vi "Bridge Lower Auto.vi"(9 "d":dbl) -> ()   [LabVIEW 2011]
uses:
  <vilib>/Rock Robotics/WPI/Solenoid/WPI_SolenoidValue.ctl
  <vilib>/Rock Robotics/WPI/Solenoid/WPI_SolenoidSetEnum.vi
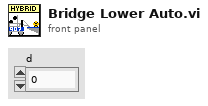
[diagram p1: front panel]
types:
  T1 = typedef "WPI_RobotDriveDevRef.ctl" = cluster{"DevStatus":errorcluster, "Motors[]":T2[], "Square Inputs":bool, "Max Output":dbl, "Isochronous":bool}
  T2 = typedef "WPI_MotorControlDeviceRef.ctl" = cluster{"DeviceStatus":errorcluster, "Type":enum16{"PWM", "CAN"}, "PWM":cluster{"Digital Module":T3, "PWM Channel":T4, "DeadBand":T5}, "CAN":cluster{"Device Number":u8, "Control Mode":T6, "Semaphore":T7, "Max Vout":dbl}, "Invert":bool, "TransformRef":T8, "InvTransformRef":T8}
  T3 = typedef "FPGA_TypedefDigitalModule.ctl" = enum16{"Digital Module 1", "Digital Module 2"}
  T4 = typedef "FPGA_DIOPWMChannel.ctl" = enum8{"PWM 1", "PWM 2", "PWM 3", "PWM 4", "PWM 5", "PWM 6", "PWM 7", "PWM 8", "PWM 9", "PWM 10", "Invalid"}
  T5 = typedef "WPI_PWMDeadband.ctl" = cluster{"Name":string, "maxPositivePwm":i32, "minPositivePwm":i32, "centerPwm":i32, "maxNegativePwm":i32, "minNegativePwm":i32, "angularRange":u16}
  T6 = typedef "WPI_CANJaguar_ControlMode.ctl" = enum8{"Percent VBus", "Current", "Speed", "Position", "Voltage"}
  T7 = typedef "Semaphore RefNum" = refnum<k1>
  T8 = typedef "WPI_PWMTransform_ConPane.ctl" = refnum<vi>
  T9 = typedef "WPI_SolenoidDevRef.ctl" = cluster{"DevStatus":errorcluster, "Solenoid Module":T10, "Forward Solenoid Channel":T11, "Reverse Solenoid Channel":T11}
  T10 = typedef "FPGA_TypedefSolenoidModule.ctl" = enum16{"Solenoid Module 1", "Solenoid Module 2"}
  T11 = typedef "WPI_SolenoidChannel.ctl" = enum8{"Solenoid 1", "Solenoid 2", "Solenoid 3", "Solenoid 4", "Solenoid 5", "Solenoid 6", "Solenoid 7", "Solenoid 8", "Invalid"}
  T12 = typedef "WPI_EncoderDevRef.ctl" = cluster{"DevStatus":errorcluster, "EncoderIndex":T13, "CounterIndex":T14, "DistancePerCount":dbl, "Decoding Type":T15}
  T13 = typedef "FPGA_EncoderIdx.ctl" = enum8{"Enc 0", "Enc 1", "Enc 2", "Enc 3", "Invalid"}
  T14 = typedef "FPGA_CounterCtrSystemIndex.ctl" = enum8{"Ctr 0", "Ctr 1", "Ctr 2", "Ctr 3", "Ctr 4", "Ctr 5", "Ctr 6", "Ctr 7", "Invalid"}
  T15 = typedef "WPI_EncoderType.ctl" = enum16{"1x", "2x", "4x"}
  T16 = typedef "WPI_SolenoidValue.ctl" = enum16{"Off", "On", "Forward", "Reverse"}
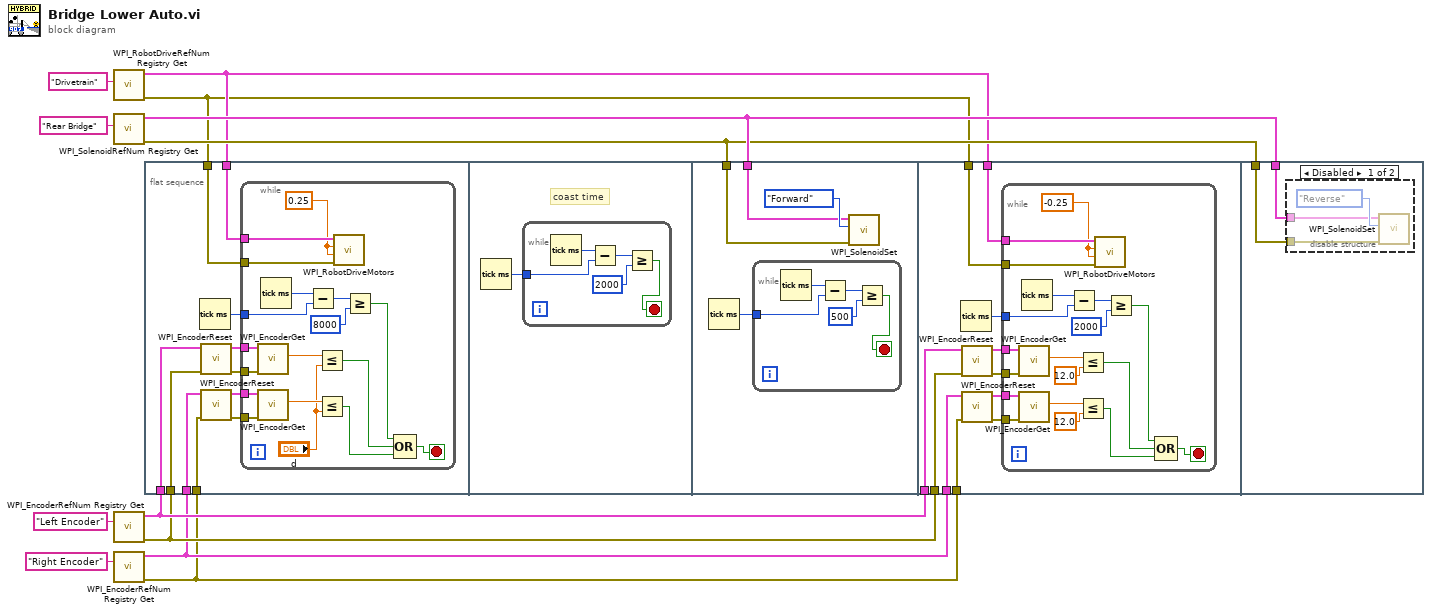
[diagram p0: block diagram]
diagram:
  n1 = call <vilib>:"WPI_RobotDriveRefNum Registry Get.vi"("refnum name"="Drivetrain") -> ("error out"=w7:errorcluster, "RobotDriveDevRef"=w8:T1)  [unwired: 9 in]
  n2 = call <vilib>:"WPI_SolenoidRefNum Registry Get.vi"("refnum name"="Rear Bridge") -> ("error out"=w9:errorcluster, "SolenoidDevRef"=w10:T9)  [unwired: 9 in]
  n3 = call <vilib>:"WPI_EncoderRefNum Registry Get.vi"("refnum name"="Left Encoder") -> ("error out"=w4:errorcluster, "EncoderDevRef"=w5:T12)  [unwired: 9 in]
  n4 = call <vilib>:"WPI_EncoderRefNum Registry Get.vi"("refnum name"="Right Encoder") -> ("error out"=w1:errorcluster, "EncoderDevRef"=w2:T12)  [unwired: 9 in]
  n5 = flat-sequence {
    tunnel: w8 -> [w22]
    tunnel: w7 -> [w21]
    tunnel: w5 -> [w19]
    tunnel: w4 -> [w20]
    tunnel: w2 -> [w14]
    tunnel: w1 -> [w13]
    tunnel: w10 -> [w49]
    tunnel: w9 -> [w48]
    tunnel: w8 -> [w61]
    tunnel: w7 -> [w62]
    tunnel: w5 -> [w60]
    tunnel: w4 -> [w59]
    tunnel: w2 -> [w58]
    tunnel: w1 -> [w57]
    tunnel: w10 -> [w88]
    tunnel: w9 -> [w87]
    frame #0 {
      n6 = Tick Count (ms)() -> (millisecond timer value=w23:u32)
      n7 = call <vilib>:"WPI_EncoderReset.vi"("error in (no error)"=w20, "EncoderDevRef"=w19) -> ("error out"=w17:errorcluster, "EncoderDevRef"=w18:T12)  [unwired: 8 in]
      n8 = call <vilib>:"WPI_EncoderReset.vi"("error in (no error)"=w13, "EncoderDevRef"=w14) -> ("error out"=w16:errorcluster, "EncoderDevRef"=w15:T12)  [unwired: 8 in]
      n9 = while {
        tunnel: w23 -> [w37]
        tunnel: w22 -> [w40]
        tunnel: w21 -> [w39]
        tunnel: w18 -> [w33]
        tunnel: w17 -> [w34]
        tunnel: w15 -> [w31]
        tunnel: w16 -> [w30]
        stop <- w29 stop-if-true
        w35 = 0.25 ("Left axis value")
        n10 = call <vilib>:"WPI_EncoderGet.vi"("error in (no error)"=w34, "EncoderDevRef"=w33) -> ("Distance"=w32:dbl)  [unwired: 4 in, 5 out]
        n11 = call <vilib>:"WPI_EncoderGet.vi"("error in (no error)"=w30, "EncoderDevRef"=w31) -> ("Distance"=w25:dbl)  [unwired: 4 in, 5 out]
        n12 = Tick Count (ms)() -> (millisecond timer value=w36:u32)
        n13 = Subtract(x=w36, y=w37) -> (x-y=w41:u32)
        n14 = Less Or Equal?(x=w32, y="d") -> (x <= y?=w27:bool)
        n15 = Less Or Equal?(x=w25, y="d") -> (x <= y?=w28:bool)
        n16 = call <vilib>:"WPI_RobotDriveMotors.vi"("error in (no error)"=w39, "RightSpeed"=w35, "LeftSpeed"=w35, "RobotDriveDevRef"=w40) -> ()  [unwired: 6 in, 2 out]
        n17 = Greater Or Equal?(x=w41, y=u32 8000) -> (x >= y?=w26:bool)
        n18 = Compound Arithmetic op=OR(w26, w27, w28) -> (w29:bool)
      }
    }
    frame #1 {
      # "coast time"
      n19 = Tick Count (ms)() -> (millisecond timer value=w42:u32)
      n20 = while {
        tunnel: w42 -> [w43]
        stop <- w45 stop-if-true
        n21 = Tick Count (ms)() -> (millisecond timer value=w44:u32)
        n22 = Subtract(x=w44, y=w43) -> (x-y=w47:u32)
        n23 = Greater Or Equal?(x=w47, y=u32 2000) -> (x >= y?=w45:bool)
      }
    }
    frame #2 {
      n24 = Tick Count (ms)() -> (millisecond timer value=w50:u32)
      n25 = while {
        tunnel: w50 -> [w52]
        stop <- w54 stop-if-true
        n26 = Tick Count (ms)() -> (millisecond timer value=w53:u32)
        n27 = Subtract(x=w53, y=w52) -> (x-y=w56:u32)
        n28 = Greater Or Equal?(x=w56, y=u32 500) -> (x >= y?=w54:bool)
      }
      n29 = call-poly <vilib>:"WPI_SolenoidSet.vi"("error in (no error)"=w48, "Value"=WPI_SolenoidValue."Forward", "SolenoidDevRef"=w49) -> ()  [unwired: 7 in, 2 out]
    }
    frame #3 {
      n30 = Tick Count (ms)() -> (millisecond timer value=w63:u32)
      n31 = call <vilib>:"WPI_EncoderReset.vi"("error in (no error)"=w59, "EncoderDevRef"=w60) -> ("error out"=w65:errorcluster, "EncoderDevRef"=w64:T12)  [unwired: 8 in]
      n32 = call <vilib>:"WPI_EncoderReset.vi"("error in (no error)"=w57, "EncoderDevRef"=w58) -> ("error out"=w66:errorcluster, "EncoderDevRef"=w67:T12)  [unwired: 8 in]
      n33 = while {
        tunnel: w63 -> [w82]
        tunnel: w61 -> [w85]
        tunnel: w62 -> [w84]
        tunnel: w64 -> [w78]
        tunnel: w65 -> [w79]
        tunnel: w67 -> [w73]
        tunnel: w66 -> [w72]
        stop <- w71 stop-if-true
        w80 = -0.25 ("Left axis value")
        n34 = call <vilib>:"WPI_EncoderGet.vi"("error in (no error)"=w79, "EncoderDevRef"=w78) -> ("Distance"=w77:dbl)  [unwired: 4 in, 5 out]
        n35 = call <vilib>:"WPI_EncoderGet.vi"("error in (no error)"=w72, "EncoderDevRef"=w73) -> ("Distance"=w74:dbl)  [unwired: 4 in, 5 out]
        n36 = Tick Count (ms)() -> (millisecond timer value=w81:u32)
        n37 = Subtract(x=w81, y=w82) -> (x-y=w86:u32)
        n38 = Less Or Equal?(x=w77, y=12.0) -> (x <= y?=w69:bool)
        n39 = Less Or Equal?(x=w74, y=12.0) -> (x <= y?=w70:bool)
        n40 = call <vilib>:"WPI_RobotDriveMotors.vi"("error in (no error)"=w84, "RightSpeed"=w80, "LeftSpeed"=w80, "RobotDriveDevRef"=w85) -> ()  [unwired: 6 in, 2 out]
        n41 = Greater Or Equal?(x=w86, y=u32 2000) -> (x >= y?=w68:bool)
        n42 = Compound Arithmetic op=OR(w68, w69, w70) -> (w71:bool)
      }
    }
    frame #4 {
      n43 = disable-structure shown="Disabled" {
        disable-tunnel: w88 -> [w90 _]
        disable-tunnel: w87 -> [w89 _]
        frame Disabled {
          n44 = call-poly <vilib>:"WPI_SolenoidSet.vi"("error in (no error)"=w89, "Value"=WPI_SolenoidValue."Reverse", "SolenoidDevRef"=w90) -> ()  [unwired: 7 in, 2 out]
        }
        frame Enabled {
        }
      }
    }
  }
